vi "StringToBool_Ctl_3.vi"(8 "error in":errorcluster, 10 "8 Bit word (str)":string) -> (0 "error out":errorcluster, 1 "Bool Out":bool[](array[boolean]), 2 "Num Out":dbl[](array[numeric]), 4 "8 Bit word (str) out":string)   [LabVIEW 2018]
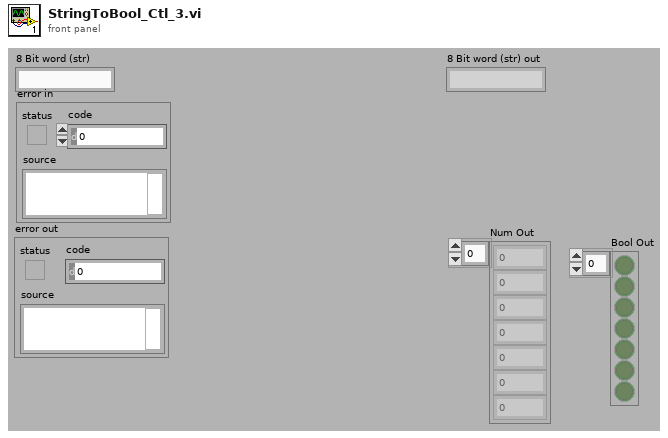
[diagram p1: front panel]
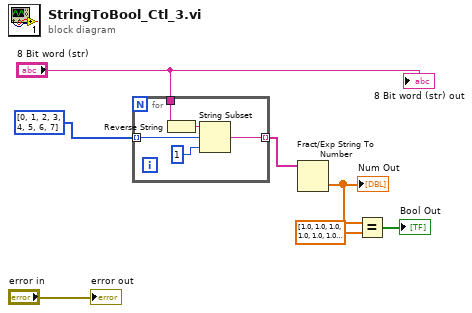
[diagram p0: block diagram]
diagram:
  n1 = for {
    tunnel: "8 Bit word (str)" -> [w12]
    tunnel: [w10] -> w5 mode=indexing
    tunnel: i32[] [0, 1, 2, 3, 4, 5, 6, 7] -> [w9] mode=indexing
    n2 = Reverse String(1:w12) -> (0:w8:string)
    n3 = String Subset(string=w8, offset (0)=w9, length (rest)=1 ("length (rest)")) -> (substring=w10:string)
  }
  n4 = Fract/Exp String To Number(string=w5) -> (number=w4:dbl[])  [unwired: 3 in, 1 out]
  "Num Out" <- w4
  n5 = Equal?(x=w4, y=dbl[] [1.0, 1.0, 1.0, 1.0, 1.0, 1.0, 1.0, 1.0]) -> (x = y?=→"Bool Out":bool[])
  "8 Bit word (str) out" <- "8 Bit word (str)"
  "error out" <- "error in"
